vi "createUsableFilename.vi"(8 "error in (no error)":errorcluster, 9 "Timestamp":timestamp, 10 "Base filename":string, 11 "Write directory":path) -> (0 "error out":errorcluster, 3 "Available file path":path)   [LabVIEW 2017]
doc: "Create a timestamped unique file in a given directory, creating the directory if necessary"
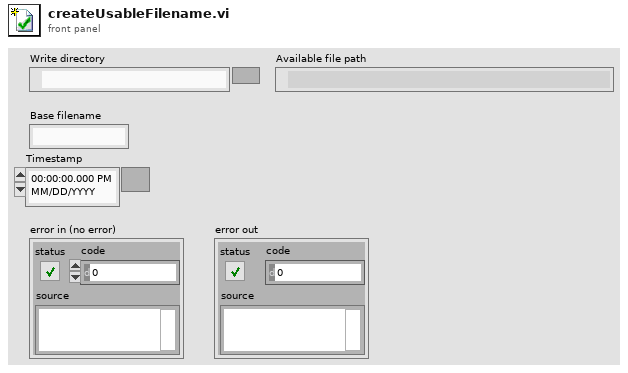
[diagram p1: front panel]
types:
  T1 = enum16{"Overwrite", "Append number", "Append date & time"}
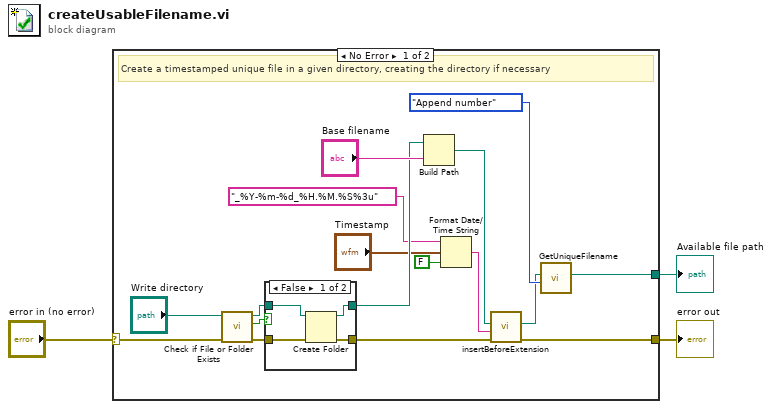
[diagram p0: block diagram]
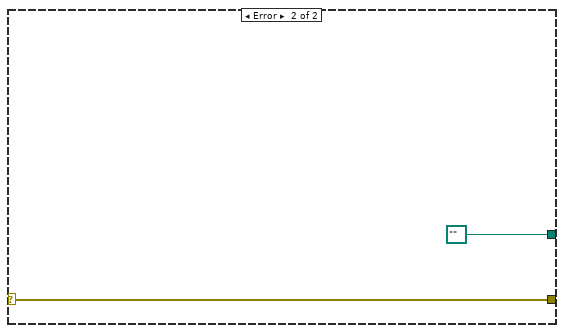
[diagram p3: hidden frame]
diagram:
  n1 = case shown="No Error" "error in (no error)" {
    selector: "error in (no error)" -> [w5 w28]
    tunnel: [w7 w28] -> w3
    tunnel: [w4 path "" ("Output path")] -> w1
    frame No Error {
      # "Create a timestamped unique file in a given directory, creating the directory if necessary"
      n2 = call <vilib>:"Check if File or Folder Exists.vi"("error in (no error)"=w5, "path"="Write directory") -> ("error out"=w17:errorcluster, "file or folder exists?"=w15:bool, "dup path"=w16:path)  [unwired: 7 in]
      n3 = case shown="False" w15 {
        tunnel: w16 -> [w24 w26]
        tunnel: w17 -> [w23 w25]
        tunnel: [w22 w25] -> w8
        tunnel: [w21 w26] -> w18
        frame False {
          n4 = Create Folder(path (use dialog)=w24, error in=w23) -> (created path=w21:path, error out=w22:errorcluster)  [unwired: 1 in, 1 out]
        }
        frame True {
        }
      }
      n5 = Build Path(base path=w18, name or relative path="Base filename") -> (appended path=w13:path)
      n6 = Format Date/Time String(time format string (%c)="_%Y-%m-%d_%H.%M.%S%3u", seconds (now)="Timestamp", UTC format=FALSE) -> (date/time string=w9:string)
      n7 = call "insertBeforeExtension.vi"("error in (no error)"=w8, "Insert"=w9, "Filepath"=w13) -> ("error out"=w7:errorcluster, "Filepath with insert"=w6:path)  [unwired: 7 in]
      n8 = call "GetUniqueFilename.vi"("Enum"=T1."Append number" ("Overwrite mode"), "Input path"=w6) -> ("Output path"=w4:path)  [unwired: 9 in]
    }
    frame Error {
    }
  }
  "error out" <- w3
  "Available file path" <- w1
